vi "ExposeInvokeMethod.vi"(0 "Expose Info in":T1, 1 "Method Name":string, 2 "Argument(s)":variant, 3 "Rsp. Type (or value to update)":variant, 4 "Require Response":bool, 5 "error in (no error)":errorcluster) -> (14 "Expose out":T1, 15 "Response":variant, 19 "error out":errorcluster)   [LabVIEW 2017]
uses:
  ExposeInfo.ctl
  C:/Code/CMCryoSysCode/Expose/COM/CSCom/CSCom/bin/Release/CSCom.dll
  COM/CSCom/CSCom/bin/Release/CSCom.dll
  ExposeMessage.ctl
  Events/ExposeMessageType.ctl
  Mapper/ExposeObjectMapNamepathData.ctl
  Mapper/ExposeMapperDataTypeEnum.ctl
  Mapper/ExposeObjectMapContainerTypeEnum.ctl
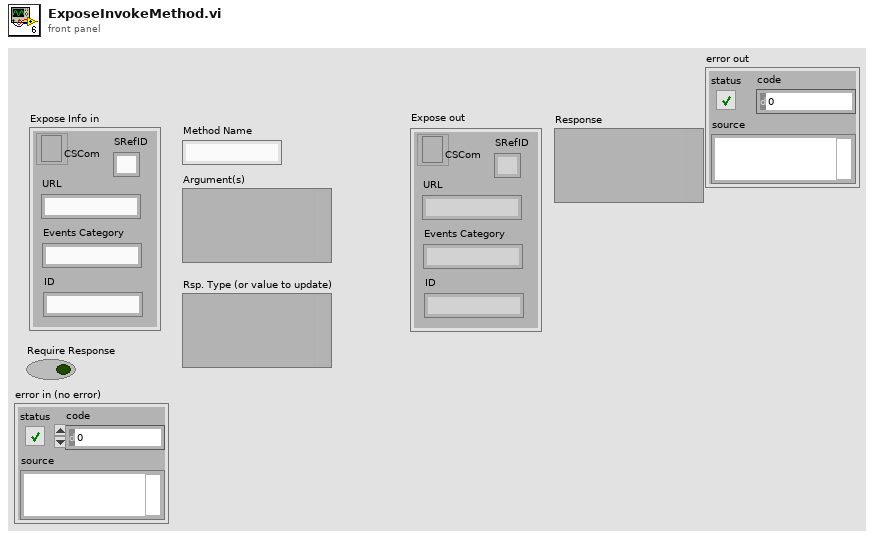
[diagram p1: front panel]
types:
  T1 = typedef "ExposeInfo.ctl" = cluster{"CSCom":refnum<k24>, "URL":string, "Events Category":string, "ID":string, "SRefID":string}
  T2 = typedef "ExposeMessage.ctl" = cluster{"Message Type":T3, "Text":string, "NamepathInfo":T4[]}
  T3 = typedef "ExposeMessageType.ctl" = i32
  T4 = typedef "ExposeObjectMapNamepathData.ctl" = cluster{"Type":T5, "Value":variant, "Namepath":string, "Container Type":T6}
  T5 = typedef "ExposeMapperDataTypeEnum.ctl" = enum16{"NotData", "int8", "byte", "int16", "uint16", "int32", "uint32", "int64", "uint64", "Single", "Double", "String", "Boolean", "Container"}
  T6 = typedef "ExposeObjectMapContainerTypeEnum.ctl" = enum16{"Value", "Array", "Waveform", "NetContainer"}
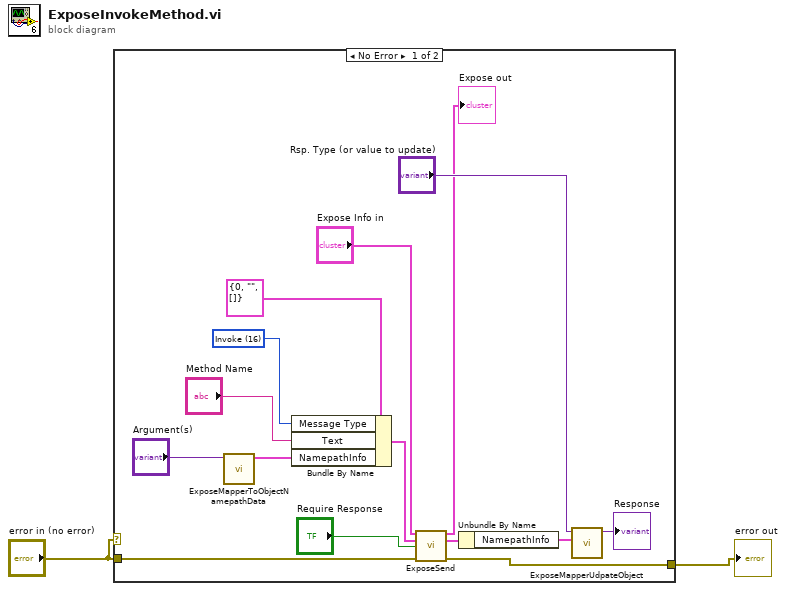
[diagram p0: block diagram]
diagram:
  n1 = case shown="No Error" "error in (no error)" {
    tunnel: "error in (no error)" -> [w4 w18]
    tunnel: [w3 w18] -> w1
    frame No Error {
      w6 = T3 16 items=["Error"=1, "Warning"=2, "Create"=4, "Destroy"=8, "Invoke"=16, "Get"=32, "Set"=64, "Response"=128] ("Message Type")
      n2 = call "ExposeMapperToObjectNamepathData.vi"("Value"="Argument(s)") -> ("Object map"=w11:T4[])  [unwired: 10 in]
      n3 = Bundle By Name(cluster=T2 {"Message Type"=0, "Text"="", "NamepathInfo"=[]} ("Message"), "Message Type"=w6, "Text"="Method Name", "NamepathInfo"=w11) -> (w12:T2)
      n4 = call "ExposeSend.vi"("Expose"="Expose Info in", "Message"=w12, "Require Response"="Require Response", "error in (no error)"=w4) -> ("Expose out"=→"Expose out":T1, "Response"=w14:T2, "error out"=w3:errorcluster)  [unwired: 9 in]
      n5 = Unbundle By Name(w14) -> ("NamepathInfo"=w15:T4[])
      n6 = call "ExposeMapperUdpateObject.vi"("Object Map"=w15, "Type (or value to update)"="Rsp. Type (or value to update)") -> ("Value"=→"Response":variant)  [unwired: 8 in, 1 out]
    }
    frame Error {
    }
  }
  "error out" <- w1
